vi "host.vi"() -> ()   [LabVIEW 2020]
uses:
  <vilib>/rvi/interface/RandomDataEmulation/nirviRandomDataOpen.vi
  <vilib>/rvi/interface/common/niFpgaCacheSessionInfoDynamic.vi
  <vilib>/Utility/error.llb/Error Cluster From Error Code.vi
  <vilib>/rvi/interface/common/niFpgaWaitOnOcc.vi
  <vilib>/rvi/errors/niLvFpgaAdjustHostInterfaceError.vi
  <vilib>/FPGAPlugInAG/Dynamic/niLvFpga_Run_Dynamic.vi
  <vilib>/FPGAPlugInAG/Dynamic/niLvFpga_Close_Dynamic.vi
  <vilib>/rvi/interface/nirviOpenFPGA/nirviOpenFPGA.xnode
  FFT.vi
  <vilib>/rvi/interface/nirviMethod/nirviMethod.xnode
  <vilib>/rvi/interface/nirviCloseFPGA/nirviCloseFPGA.xnode
  <vilib>/rvi/errors/niLvFpgaMergeErrorWithErrorCode.vi
  <vilib>/FPGAPlugInAG/Dynamic/niLvFpga_ReadFifo_Dynamic.vi
  <vilib>/Analysis/NI_AALPro.lvlib
  <vilib>/FPGAPlugInAG/Dynamic/niLvFpga_ConfigureFifo_Dynamic.vi
  <vilib>/FPGAPlugInAG/Dynamic/niLvFpga_StartFifo_Dynamic.vi
  <vilib>/FPGAPlugInAG/Dynamic/niLvFpga_WriteFifo_Dynamic.vi
panel:
  out "truth/restored/final":dbl[][](graph)
  out "final signal trend add":dbl[](graph)
  out "restored   trend add":dbl[](graph)
  out "final signal":fxp<+/-,32,16>[](array[numeric])
  out "final signal":dbl[](graph)
  out "final signal":i32
  out "restored signal":dbl[](graph)
  out "restored signal size":i32
  out "restored signal":fxp<+/-,32,15>[](array[numeric])
  out "phase 2 index":dbl[](graph)
  out "phase 2 size":i32
  out "mag 2 index":dbl[](graph)
  out "mag 2 size":i32
  out "phase 2":fxp<+/-,32,15>[](array[numeric])
  out "mag 2":fxp<+/-,32,15>[](array[numeric])
  out "frequency index":dbl[](graph)
  out "frequency size":i32
  out "freq":fxp<+/-,32,15>[](array[numeric])
  out "magnitude":dbl[](graph)
  out "phase":dbl[](graph)
  out "phase size":i32
  out "mag size":i32
  out "phase":fxp<+/-,32,15>[](array[numeric])
  out "magnitude":fxp<+/-,32,15>[](array[numeric])
  out "Actual Depth":u32
  out "host to target":u32
  out "signal_target_to_host_fixed size(s)":i32
  out "target to host 1":u32
  out "signal target to host":dbl[][](graph)
  out "signal_target_to_host_fixed":fxp<+/-,24,7>[](array[numeric])
  out "Array 2":fxp<+/-,24,7>[](array[numeric])
  out "detrend acc":dbl[](graph)
  out "samples":i32
  out "input signal":T1(graph)
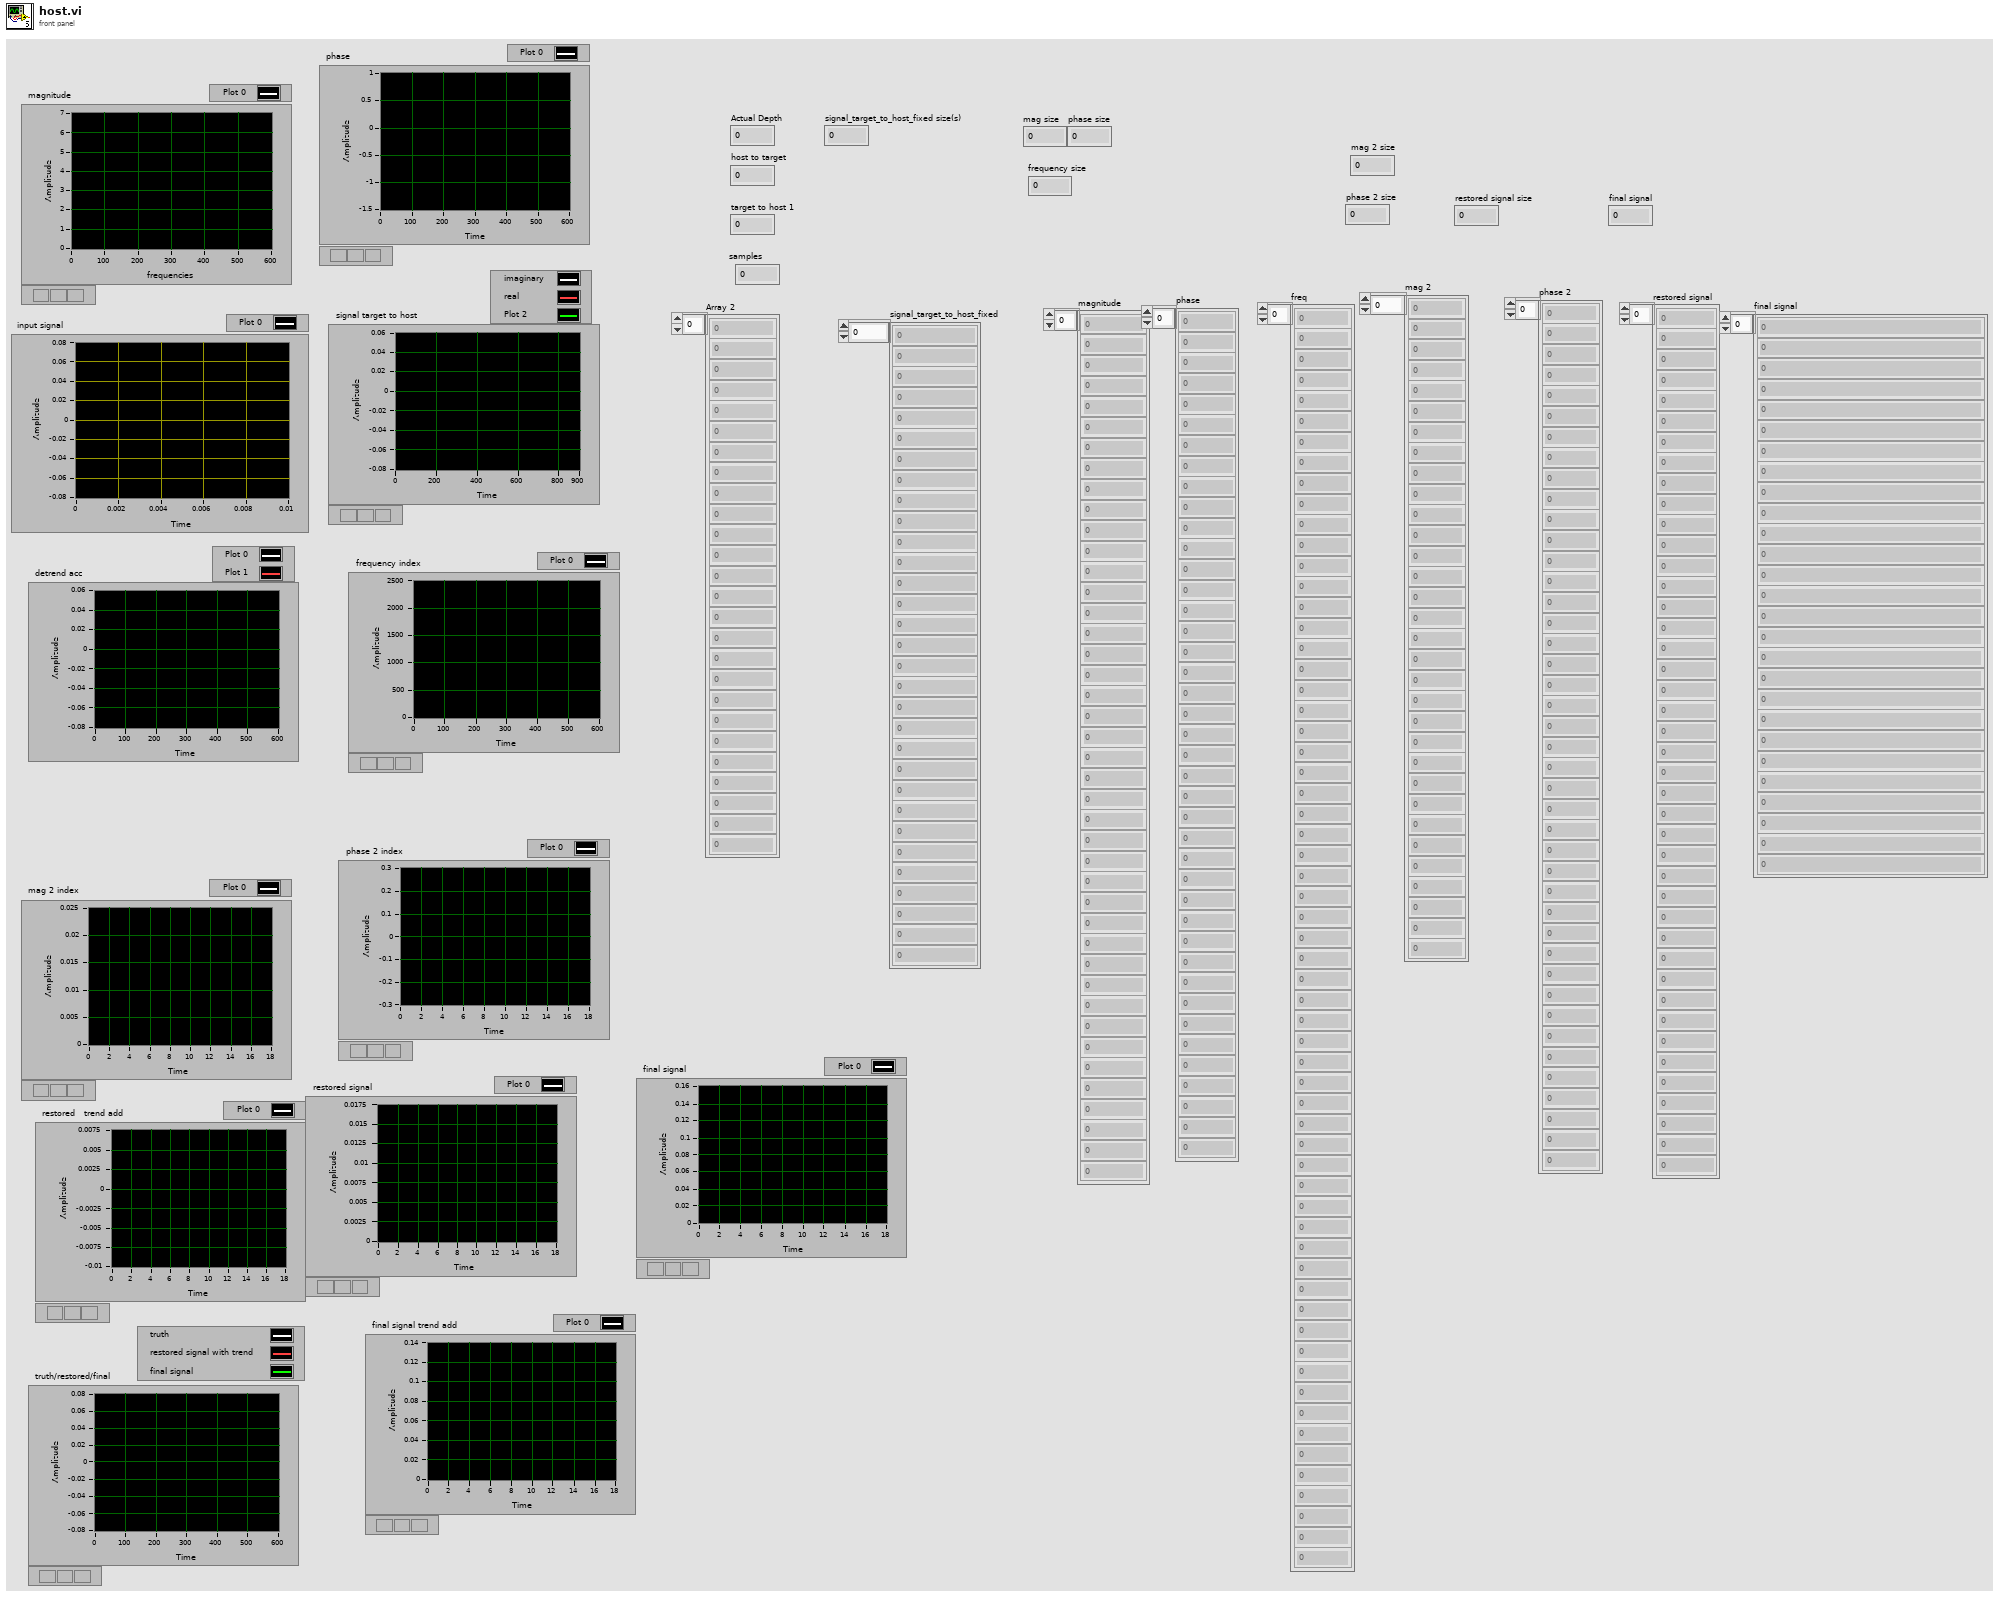
[diagram p1: front panel]
types:
  T1 = cluster{"array type (2D Dbl)":dbl[], "array type (2D Dbl)":dbl[]}
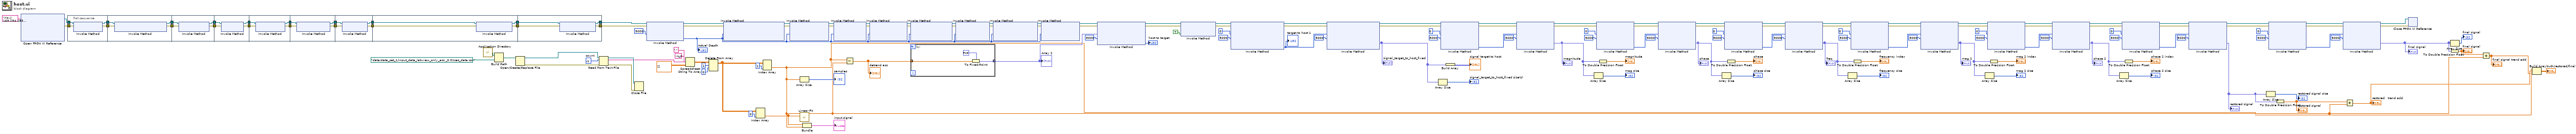
[diagram p0: block diagram]
diagram:
  w155 = -1  # count
  n1 = xnode "Open FPGA VI Reference"("resource name"=tag "rio://169.254.183.73/RIO0") -> ("FPGA VI Reference Out"=w125:refnum<k20>, "error out"=w124:errorcluster)  [unwired: 1 in]
  n2 = flat-sequence {
    tunnel: w125 -> [w168]
    tunnel: w124 -> [w167]
    tunnel: [w166] -> w26
    tunnel: [w165] -> w25
    tunnel: w26 -> [w172]
    tunnel: w25 -> [w171]
    tunnel: [w170] -> w24
    tunnel: [w169] -> w23
    tunnel: w24 -> [w176]
    tunnel: w23 -> [w175]
    tunnel: [w174] -> w22
    tunnel: [w173] -> w21
    tunnel: w22 -> [w180]
    tunnel: w21 -> [w179]
    tunnel: [w178] -> w20
    tunnel: [w177] -> w19
    tunnel: w20 -> [w184]
    tunnel: w19 -> [w183]
    tunnel: [w182] -> w18
    tunnel: [w181] -> w17
    tunnel: w18 -> [w188]
    tunnel: w17 -> [w187]
    tunnel: [w186] -> w16
    tunnel: [w185] -> w15
    tunnel: w16 -> [w192]
    tunnel: w15 -> [w191]
    tunnel: [w190] -> w14
    tunnel: [w189] -> w13
    tunnel: w14 -> [w195]
    tunnel: w13 -> [w196]
    tunnel: [w194] -> w12
    tunnel: [w193] -> w11
    tunnel: w12 -> [w200]
    tunnel: w11 -> [w199]
    tunnel: [w198] -> w10
    tunnel: [w197] -> w9
    frame #0 {
      n3 = xnode "Invoke Method"("FPGA VI Reference In"=w168, "error in"=w167) -> ("FPGA VI Reference Out"=w166:refnum<k20>, "error out"=w165:errorcluster)
    }
    frame #1 {
      n4 = xnode "Invoke Method"("FPGA VI Reference In"=w172, "error in"=w171) -> ("FPGA VI Reference Out"=w170:refnum<k20>, "error out"=w169:errorcluster)
    }
    frame #2 {
      n5 = xnode "Invoke Method"("FPGA VI Reference In"=w176, "error in"=w175) -> ("FPGA VI Reference Out"=w174:refnum<k20>, "error out"=w173:errorcluster)
    }
    frame #3 {
      n6 = xnode "Invoke Method"("FPGA VI Reference In"=w180, "error in"=w179) -> ("FPGA VI Reference Out"=w178:refnum<k20>, "error out"=w177:errorcluster)
    }
    frame #4 {
      n7 = xnode "Invoke Method"("FPGA VI Reference In"=w184, "error in"=w183) -> ("FPGA VI Reference Out"=w182:refnum<k20>, "error out"=w181:errorcluster)
    }
    frame #5 {
      n8 = xnode "Invoke Method"("FPGA VI Reference In"=w188, "error in"=w187) -> ("FPGA VI Reference Out"=w186:refnum<k20>, "error out"=w185:errorcluster)
    }
    frame #6 {
      n9 = xnode "Invoke Method"("FPGA VI Reference In"=w192, "error in"=w191) -> ("FPGA VI Reference Out"=w189:refnum<k20>, "error out"=w190:errorcluster)
    }
    frame #7 {
      n10 = xnode "Invoke Method"("FPGA VI Reference In"=w196, "error in"=w195) -> ("FPGA VI Reference Out"=w194:refnum<k20>, "error out"=w193:errorcluster)
    }
    frame #8 {
      n11 = xnode "Invoke Method"("FPGA VI Reference In"=w200, "error in"=w199) -> ("FPGA VI Reference Out"=w198:refnum<k20>, "error out"=w197:errorcluster)
    }
  }
  n12 = call <vilib>:"Application Directory.vi"() -> ("Application Directory"=w159:path)
  n13 = Build Path(base path=w159, name or relative path=path "data/data_set_1/input_data_labview_only_acc _0.01sec_data.csv" ("default name")) -> (appended path=w158:path)
  n14 = Open/Create/Replace File(file path (use dialog)=w158) -> (refnum out=w163:refnum<file>, error out=w164:errorcluster)  [unwired: 5 in, 1 out]
  n15 = Read from Text File(file (use dialog)=w163, count=w155, error in=w164) -> (refnum out=w162:refnum<file>, text=w160:string, error out=w161:errorcluster)  [unwired: 1 in, 1 out]
  n16 = Close File(refnum=w162, error in=w161) -> ()  [unwired: 2 out]
  n17 = xnode "Invoke Method"("FPGA VI Reference In"=w10, "error in"=w9, "Requested Depth"=u32 5000) -> ("FPGA VI Reference Out"=w123:refnum<k20>, "error out"=w122:errorcluster, "Actual Depth"=w31:u32)
  "Actual Depth" <- w31
  n18 = Spreadsheet String To Array(delimiter (Tab)=",", format string="%f", spreadsheet string=w160, array type (2D Dbl)=dbl[][] []) -> (array=w152:dbl[][])
  n19 = Delete From Array(array=w152, length=1, index (row)=0) -> (array with subset deleted=w147:dbl[][])  [unwired: 1 in, 1 out]
  n20 = xnode "Invoke Method"("FPGA VI Reference In"=w123, "error in"=w122, "Requested Depth"=w31) -> ("FPGA VI Reference Out"=w121:refnum<k20>, "error out"=w120:errorcluster)  [unwired: 1 out]
  n21 = Index Array(array=w147, index (col)=0 ("disabled index (col)")) -> (element=w5:dbl[])  [unwired: 1 in]
  n22 = Index Array(array=w147, index (col)=1 ("disabled index (col)")) -> (element=w2:dbl[])  [unwired: 1 in]
  n23 = xnode "Invoke Method"("FPGA VI Reference In"=w121, "error in"=w120, "Requested Depth"=w31) -> ("FPGA VI Reference Out"=w119:refnum<k20>, "error out"=w118:errorcluster)  [unwired: 1 out]
  n24 = Array Size(array=w2) -> (size(s)=→"samples":i32)
  n25 = call <vilib>:"Linear Fit.vi"("Y"=w2, "X"=w5) -> ("Best Linear Fit"=w6:dbl[])  [unwired: 9 in, 4 out]
  n26 = Bundle("array type (2D Dbl)"=w5, "array type (2D Dbl)"=w2) -> (→"input signal":T1)  [unwired: 1 in]
  n27 = xnode "Invoke Method"("FPGA VI Reference In"=w119, "error in"=w118, "Requested Depth"=w31) -> ("FPGA VI Reference Out"=w85:refnum<k20>, "error out"=w84:errorcluster)  [unwired: 1 out]
  n28 = Subtract(x=w2, y=w6) -> (x-y=w139:dbl[])
  "detrend acc" <- w139
  n29 = xnode "Invoke Method"("FPGA VI Reference In"=w85, "error in"=w84, "Requested Depth"=w31) -> ("FPGA VI Reference Out"=w61:refnum<k20>, "error out"=w60:errorcluster)  [unwired: 1 out]
  n30 = xnode "Invoke Method"("FPGA VI Reference In"=w61, "error in"=w60, "Requested Depth"=w31) -> ("FPGA VI Reference Out"=w63:refnum<k20>, "error out"=w62:errorcluster)  [unwired: 1 out]
  n31 = for {
    tunnel: [w202] -> w138 mode=indexing
    tunnel: w139 -> [w201] mode=indexing
    n32 = To Fixed-Point(fixed-point type=fxp<+/-,24,7> 0.0 ("f"), number=w201) -> (fixed-point=w202:fxp<+/-,24,7>)
  }
  "Array 2" <- w138
  n33 = xnode "Invoke Method"("FPGA VI Reference In"=w63, "error in"=w62, "Requested Depth"=w31) -> ("FPGA VI Reference Out"=w46:refnum<k20>, "error out"=w45:errorcluster)  [unwired: 1 out]
  n34 = xnode "Invoke Method"("FPGA VI Reference In"=w46, "error in"=w45, "Requested Depth"=w31) -> ("FPGA VI Reference Out"=w30:refnum<k20>, "error out"=w29:errorcluster)  [unwired: 1 out]
  n35 = xnode "Invoke Method"("FPGA VI Reference In"=w30, "error in"=w29, "Requested Depth"=w31) -> ("FPGA VI Reference Out"=w28:refnum<k20>, "error out"=w27:errorcluster)  [unwired: 1 out]
  n36 = xnode "Invoke Method"("FPGA VI Reference In"=w28, "error in"=w27, "Data"=w138, "Timeout (ms)"=5000) -> ("FPGA VI Reference Out"=w144:refnum<k20>, "error out"=w143:errorcluster, "Empty Elements Remaining"=→"host to target":u32)
  n37 = xnode "Invoke Method"("FPGA VI Reference In"=w144, "error in"=w143, "Wait Until Done (F)"=TRUE) -> ("FPGA VI Reference Out"=w129:refnum<k20>, "error out"=w128:errorcluster)
  n38 = xnode "Invoke Method"("FPGA VI Reference In"=w129, "error in"=w128, "Number of Elements"=u32 0, "Timeout (ms)"=5000) -> ("FPGA VI Reference Out"=w137:refnum<k20>, "error out"=w136:errorcluster, "Elements Remaining"=w135:u32)  [unwired: 1 out]
  "target to host 1" <- w135
  n39 = xnode "Invoke Method"("FPGA VI Reference In"=w137, "error in"=w136, "Number of Elements"=w135, "Timeout (ms)"=5000) -> ("FPGA VI Reference Out"=w100:refnum<k20>, "error out"=w99:errorcluster, "Data"=w131:fxp<+/-,24,7>[])  [unwired: 1 out]
  "signal_target_to_host_fixed" <- w131
  n40 = Array Size(array=w131) -> (size(s)=→"signal_target_to_host_fixed size(s)":i32)
  n41 = xnode "Invoke Method"("FPGA VI Reference In"=w100, "error in"=w99, "Number of Elements"=u32 0, "Timeout (ms)"=5000) -> ("FPGA VI Reference Out"=w114:refnum<k20>, "error out"=w113:errorcluster, "Elements Remaining"=w108:u32)  [unwired: 1 out]
  n42 = Build Array(w131) -> (→"signal target to host":fxp<+/-,24,7>[][])
  n43 = xnode "Invoke Method"("FPGA VI Reference In"=w114, "error in"=w113, "Number of Elements"=w108, "Timeout (ms)"=5000) -> ("FPGA VI Reference Out"=w112:refnum<k20>, "error out"=w111:errorcluster, "Data"=w98:fxp<+/-,32,16>[])  [unwired: 1 out]
  "magnitude" <- w98
  n44 = Array Size(array=w98) -> (size(s)=→"mag size":i32)
  n45 = xnode "Invoke Method"("FPGA VI Reference In"=w112, "error in"=w111, "Number of Elements"=u32 0, "Timeout (ms)"=5000) -> ("FPGA VI Reference Out"=w110:refnum<k20>, "error out"=w109:errorcluster, "Elements Remaining"=w104:u32)  [unwired: 1 out]
  n46 = To Double Precision Float(number=w98) -> (double precision float=→"magnitude":dbl[])
  n47 = xnode "Invoke Method"("FPGA VI Reference In"=w110, "error in"=w109, "Number of Elements"=w104, "Timeout (ms)"=5000) -> ("FPGA VI Reference Out"=w87:refnum<k20>, "error out"=w86:errorcluster, "Data"=w97:fxp<+/-,16,2>[])  [unwired: 1 out]
  "phase" <- w97
  n48 = Array Size(array=w97) -> (size(s)=→"phase size":i32)
  n49 = xnode "Invoke Method"("FPGA VI Reference In"=w87, "error in"=w86, "Number of Elements"=u32 0, "Timeout (ms)"=5000) -> ("FPGA VI Reference Out"=w96:refnum<k20>, "error out"=w95:errorcluster, "Elements Remaining"=w92:u32)  [unwired: 1 out]
  n50 = To Double Precision Float(number=w97) -> (double precision float=→"phase":dbl[])
  n51 = xnode "Invoke Method"("FPGA VI Reference In"=w96, "error in"=w95, "Number of Elements"=w92, "Timeout (ms)"=5000) -> ("FPGA VI Reference Out"=w71:refnum<k20>, "error out"=w70:errorcluster, "Data"=w89:fxp<+/-,32,16>[])  [unwired: 1 out]
  "freq" <- w89
  n52 = Array Size(array=w89) -> (size(s)=→"frequency size":i32)
  n53 = xnode "Invoke Method"("FPGA VI Reference In"=w71, "error in"=w70, "Number of Elements"=u32 0, "Timeout (ms)"=5000) -> ("FPGA VI Reference Out"=w83:refnum<k20>, "error out"=w82:errorcluster, "Elements Remaining"=w79:u32)  [unwired: 1 out]
  n54 = To Double Precision Float(number=w89) -> (double precision float=→"frequency index":dbl[])
  n55 = xnode "Invoke Method"("FPGA VI Reference In"=w83, "error in"=w82, "Number of Elements"=w79, "Timeout (ms)"=5000) -> ("FPGA VI Reference Out"=w69:refnum<k20>, "error out"=w68:errorcluster, "Data"=w65:fxp<+/-,32,16>[])  [unwired: 1 out]
  "mag 2" <- w65
  n56 = Array Size(array=w65) -> (size(s)=→"mag 2 size":i32)
  n57 = xnode "Invoke Method"("FPGA VI Reference In"=w69, "error in"=w68, "Number of Elements"=u32 0, "Timeout (ms)"=5000) -> ("FPGA VI Reference Out"=w77:refnum<k20>, "error out"=w76:errorcluster, "Elements Remaining"=w73:u32)  [unwired: 1 out]
  n58 = To Double Precision Float(number=w65) -> (double precision float=→"mag 2 index":dbl[])
  n59 = xnode "Invoke Method"("FPGA VI Reference In"=w77, "error in"=w76, "Number of Elements"=w73, "Timeout (ms)"=5000) -> ("FPGA VI Reference Out"=w52:refnum<k20>, "error out"=w49:errorcluster, "Data"=w64:fxp<+/-,16,2>[])  [unwired: 1 out]
  "phase 2" <- w64
  n60 = Array Size(array=w64) -> (size(s)=→"phase 2 size":i32)
  n61 = xnode "Invoke Method"("FPGA VI Reference In"=w52, "error in"=w49, "Number of Elements"=u32 0, "Timeout (ms)"=5000) -> ("FPGA VI Reference Out"=w51:refnum<k20>, "error out"=w50:errorcluster, "Elements Remaining"=w54:u32)  [unwired: 1 out]
  n62 = To Double Precision Float(number=w64) -> (double precision float=→"phase 2 index":dbl[])
  n63 = xnode "Invoke Method"("FPGA VI Reference In"=w51, "error in"=w50, "Number of Elements"=w54, "Timeout (ms)"=5000) -> ("FPGA VI Reference Out"=w38:refnum<k20>, "error out"=w37:errorcluster, "Data"=w47:fxp<+/-,64,18>[])  [unwired: 1 out]
  "restored signal" <- w47
  n64 = Array Size(array=w47) -> (size(s)=→"restored signal size":i32)
  n65 = xnode "Invoke Method"("FPGA VI Reference In"=w38, "error in"=w37, "Number of Elements"=u32 0, "Timeout (ms)"=5000) -> ("FPGA VI Reference Out"=w41:refnum<k20>, "error out"=w40:errorcluster, "Elements Remaining"=w34:u32)  [unwired: 1 out]
  n66 = To Double Precision Float(number=w47) -> (double precision float=w8:dbl[])
  "restored signal" <- w8
  n67 = xnode "Invoke Method"("FPGA VI Reference In"=w41, "error in"=w40, "Number of Elements"=w34, "Timeout (ms)"=5000) -> ("FPGA VI Reference Out"=w36:refnum<k20>, "error out"=w35:errorcluster, "Data"=w32:fxp<+/-,32,16>[])  [unwired: 1 out]
  "final signal" <- w32
  n68 = Add(x=w8, y=w6) -> (x+y=w3:dbl[])
  "restored   trend add" <- w3
  n69 = xnode "Close FPGA VI Reference"("FPGA VI Reference In"=w36, "error in"=w35) -> ()  [unwired: 1 out]
  n70 = Array Size(array=w32) -> (size(s)=→"final signal":i32)
  n71 = To Double Precision Float(number=w32) -> (double precision float=w7:dbl[])
  "final signal" <- w7
  n72 = Add(x=w7, y=w6) -> (x+y=w1:dbl[])
  "final signal trend add" <- w1
  n73 = Build Array(w2, w3, w1) -> (→"truth/restored/final":dbl[][])
